vi "SSL Vision Log Player.vi"() -> ()   [LabVIEW 2017]
uses:
  SSL Referee Game Status.ctl
  GUI/IA Robot Line Display.ctl
  Intel/Functions Enum.ctl
  Filters/Estimadores.ctl
  Control/SSL Data Control.ctl
  Control/SSL UDP Address.ctl
  Control/File Player.ctl
  Intel/Command Enum.ctl
  Test/TestModule.ctl
  Util/Select None or Robot.ctl
  DrawTargets.ctl
  Select Personalitys.ctl
  Util/Select Auto None or Robot.ctl
  Intel/AI Parameters.ctl
  grSim/grSim RobotReplacement.ctl
  grSim/grSim_BallReplacement.ctl
  SSL/SSL Field State.ctl
  SSL Detection Frame.ctl
  SSL Detection Robot.ctl
  <vilib>/Analysis/Matrix/Datatypes/RealMatrix.ctl
  SSL Detection Ball.ctl
  <extravilib>/ChannelInstances/Lossy Stream-t'AI Input.ctl'/Read With Abort.vi
  <extravilib>/ChannelInstances/Lossy Stream-a[.](u8)/Read With Abort.vi
  <extravilib>/ChannelInstances/Lossy Stream-t'SSL Referee Game Status.ctl'/Write With Abort.vi
  <extravilib>/ChannelInstances/Lossy Stream-t'SSL Field State.ctl'/Write With Abort.vi
  <extravilib>/ChannelInstances/Lossy Stream-t'SSL Field State.ctl'/Read With Abort.vi
  <extravilib>/ChannelInstances/Lossy Stream-a[.](i32)/Write With Abort.vi
  <extravilib>/ChannelInstances/Lossy Stream-t'SSL Referee Game Status.ctl'/Read With Abort.vi
  <extravilib>/ChannelInstances/Lossy Stream-t'AI Input.ctl'/Write With Abort.vi
  <extravilib>/ChannelInstances/Lossy Stream-t'AI Input.ctl'/EndpointRead.vi
  <extravilib>/ChannelInstances/Lossy Stream-a[.](u8)/EndpointRead.vi
  <extravilib>/ChannelInstances/Lossy Stream-t'SSL Referee Game Status.ctl'/Endpoint.vi
  <extravilib>/ChannelInstances/Lossy Stream-t'SSL Field State.ctl'/Endpoint.vi
  <extravilib>/ChannelInstances/Lossy Stream-t'SSL Field State.ctl'/EndpointRead.vi
  <extravilib>/ChannelInstances/Lossy Stream-a[.](i32)/Endpoint.vi
  <extravilib>/ChannelInstances/Lossy Stream-t'SSL Referee Game Status.ctl'/EndpointRead.vi
  <extravilib>/ChannelInstances/Lossy Stream-t'AI Input.ctl'/Endpoint.vi
  <extravilib>/ChannelInstances/Lossy Stream-a[.](u8)/Instantiate.vi
  <extravilib>/ChannelInstances/Lossy Stream-a[.](u8)/)Channel.vi
  <resource>/ChannelSupport/_ChannelSupport/WaitIfNeeded.vi
  <extravilib>/ChannelInstances/Lossy Stream-t'AI Input.ctl'/Instantiate.vi
  <extravilib>/ChannelInstances/Lossy Stream-t'SSL Field State.ctl'/Instantiate.vi
  <extravilib>/ChannelInstances/Lossy Stream-t'AI Input.ctl'/)Channel.vi
  <extravilib>/ChannelInstances/Lossy Stream-t'SSL Field State.ctl'/)Channel.vi
  <extravilib>/ChannelInstances/Lossy Stream-a[.](i32)/Instantiate.vi
  Util/PreviousState.vi
  <extravilib>/ChannelInstances/Lossy Stream-t'SSL Referee Game Status.ctl'/Instantiate.vi
  <extravilib>/ChannelInstances/Lossy Stream-t'SSL Referee Game Status.ctl'/)Channel.vi
  <extravilib>/ChannelInstances/Lossy Stream-a[.](i32)/)Channel.vi
  <extravilib>/ChannelInstances/Lossy Stream-t'SSL Referee Game Status.ctl'.lvlib
  <extravilib>/ChannelInstances/Lossy Stream-t'AI Input.ctl'.lvlib
  <extravilib>/ChannelInstances/Lossy Stream-t'SSL Field State.ctl'.lvlib
  <extravilib>/ChannelInstances/Lossy Stream-a[.](u8).lvlib
  <vilib>/Analysis/Matrix/NI_Matrix.lvlib
  <extravilib>/ChannelInstances/Lossy Stream-a[.](i32).lvlib
panel:
  out "error IO":errorcluster
  out "Vector Flags":cluster{"id":dbl, "flag":bool}[](array[cluster])
  in  "grid y":dbl format="%#_13g"
  in  "grid x":dbl format="%#_13g"
  out "kick error":dbl
  in  "Pinned":T1={"Attc"="Auto", "Strk"="Auto", "Def"="Auto"}
  in  "Draw Targets?":T3={"Attacker"=TRUE, "Striker"=TRUE, "Goalie"=TRUE, "Defender"=TRUE, "kick"=TRUE, "Est Ball"=TRUE, "Est Robot"=FALSE}
  in  "SSL Data":T4={"Modo"=TRUE, "SSL UDP RX"={"Port:"=10020, "Server IP:"="224.5.23.2", "Local IP:"="", "RX"=TRUE}, "RefBox UDP RX"={"Port:"=10003, "Server IP:"="224.5.23.1", "Local IP:"="", "RX"=TRUE}, "Reprodução de Arquivo"={"file path (use dialog)"=path "E:/Media/2016-07-01_cmdragons_immortals.log", "size (in bytes)"=0, "offset (in bytes)"=0, "Slide"=0.0, "Play"=FALSE, "Time Stamp"=timestamp(0 s since 1904-01-01), "Playing"=FALSE}, "SSL UDP SOS RX "={"Port:"=10030, "Server IP:"="224.5.23.2", "Local IP:"="", "RX"=TRUE}} {"Reprodução de Arquivo"."Time Stamp" format="%<%.3X %x>T"; "Reprodução de Arquivo"."Slide" min=0 max=1 scale=0.0..1.0; "Reprodução de Arquivo"."offset (in bytes)" format="%.3p"; "Reprodução de Arquivo"."size (in bytes)" format="%.3p"}
  out "error out 5":errorcluster
  out "error out 3":errorcluster
  out "Pass":bool
  out "IA command":T7
  in  "ignora esquerda?":bool
  in  "ignora lado?":bool
  in  "atacando ao contrário?":bool
  in  "Defense stretch":i32=300
  in  "Defense radius":i32=460
  in  "Estimador":T8=enum."Kalman"
  out "Role Playing \nFPS":dbl
  out "Total Delay":dbl format="%#.5g"
  in  "Goalie":string(combo)="0"
  in  "Command":string(combo)="Auto"
  in  "Time":enum16{"Azul", "Amarelo"}(ring) caption="Enum"
  in  "Lado":enum16{"Esquerdo", "Direito"}(ring) caption="Enum"
  in  "Role Decisor":enum16{"Simple Role Decisor", "No Role Decisor"}(ring)
  out "bot velocity":dbl(graph)
  out "ball":dbl(graph)
  in  "test module":T9={"Goto"="None", "ZigZag 0"="None", "Kicker"="None", "Vel_kick"=100.0, "Kick"=FALSE, "Modo Teste?"=FALSE, "GoTo point"=[], "zigzag points"=[{"x"=666.0, "y"=0.0}, {"x"=-666.0, "y"=0.0}], "robot id vel"=5, "Dribble"=FALSE, "Gravando"=FALSE, "output xy"=0.0, "output angle"=0.0, "angle zigzag"=0.0}
  in  "Tab Control":enum32{"RX Info", "TX info", "AI Parameters"}(tab)
  out "GUI Robot Array":T11[](array[typedef])
  out "Game Status":T13={"Stage"="Normal First Half Pre", "Command"="Stop", "Time Left"=0.0, "Yellow Team"="", "Blue Team"="", "Yellow Score"=0, "Blue Score"=0, "Yellow Red Cards"=0, "Blue Red Cards"=0, "Yellow Yellow Cards"=0, "Blue Yellow Cards"=0, "Yellow Timeouts Left"=0, "Blue Timeouts Left"=0, "Yellow Timeout Remaining"=0.0, "Blue Timeout Remaining"=0.0, "Yellow Goalie Id"=0, "Blue Goalie Id"=0, "Time"=timestamp(2082758400 s since 1904-01-01)} {"Time" format="%<%.3X %x>T"; "Blue Timeout Remaining" format="%<%M:%S>t"; "Yellow Timeout Remaining" format="%<%M:%S>t"; "Time Left" format="%<%M:%S>t"}
  in  "Serial TX":bool
  in  "UDP TX":bool=TRUE
  in  "Address:":string="127.0.0.1"
  in  "Port:":u16=20011
  in  "Porta:":refnum<visa-resource-name>
  out "Comm FPS":dbl
  in  "replace active":bool
  in  "grSim replacement":cluster{"robots":T14[], "ball":T15}={"robots"=[{"x"=0.0, "y"=-450.0, "dir"=0.0, "yellowteam"=FALSE, "id"=0}, {"x"=0.0, "y"=-270.0, "dir"=0.0, "yellowteam"=FALSE, "id"=1}, {"x"=0.0, "y"=-90.0, "dir"=0.0, "yellowteam"=FALSE, "id"=2}, {"x"=0.0, "y"=90.0, "dir"=0.0, "yellowteam"=FALSE, "id"=3}, {"x"=0.0, "y"=270.0, "dir"=0.0, "yellowteam"=FALSE, "id"=4}, {"x"=0.0, "y"=450.0, "dir"=0.0, "yellowteam"=FALSE, "id"=5}], "ball"={"x"=0.0, "y"=0.0, "vx"=0.0, "vy"=0.0}}
  in  "AI Parameters":T16={"GotoKick"={"Dist do cone a frente"=0.0, "attacker farback"=1000.0, "Perto"=300.0, "min dist to kick"=120.0, "kick eps"=0.1, "Time to transition"=0.3}, "Attacker"={"CC chute"=0.55, "CC passe"=0.4, "Kick Force"=100.0, "D ball-robot Kick"=250.0, "D ball-robot Pass"=350.0}, "Defender"={"D max"=1700.0, "Vel p/ robô av"=3.0, "Kick Force"=100.0, "D atk-def"=400.0, "D farback"=300.0}, "Timeout"={"Field/v in x"=6.0, "Dist Robots"=300, "Dist up in y"=300}, "Pose Striker"={"dist"=650.0, "Numeric"=-4.0, "dist 2"=650.0}, "Dist Stop"=300.0, "Distance when ball out"=200, "D central gap "=125.0, "T pass"=5.0, "Force ++"=100.0, "range kick"=50.0, "Chute alto"=TRUE, "Marcador novo"=TRUE} {"D central gap" format="%#_13g"; "Dist Stop" format="%#_13g"; "Pose Striker"."Numeric" format="%#_13g"; "Defender"."Kick Force" format="%#_13g"; "Defender"."Vel p/ robô av" format="%#_13g"; "Attacker"."D ball-robot Kick" format="%#_13g"; "Attacker"."Kick Force" format="%#_13g"; "Attacker"."CC passe" format="%#_13g"; "Attacker"."CC chute" format="%#_13g"; "GotoKick"."min dist to kick" format="%#_13g"; "GotoKick"."Perto" format="%#_13g"; "GotoKick"."attacker farback" format="%#_13g"; "GotoKick"."Dist do cone a frente" format="%#_13g"}
  in  "Dist posse":dbl=220.0
  in  "Tol ang posse":dbl=0.3
  in  "Dist Toque":dbl=130.0
  in  "Qtd Min p/ Stk":dbl=2.0
  # "UDP"
  # "LOG"
  # "Score"
  # "Red Cards"
  # "Yellow Cards"
  # "Timeouts Left"
  # "Timeout Remaining"
  # "Goalie ID"
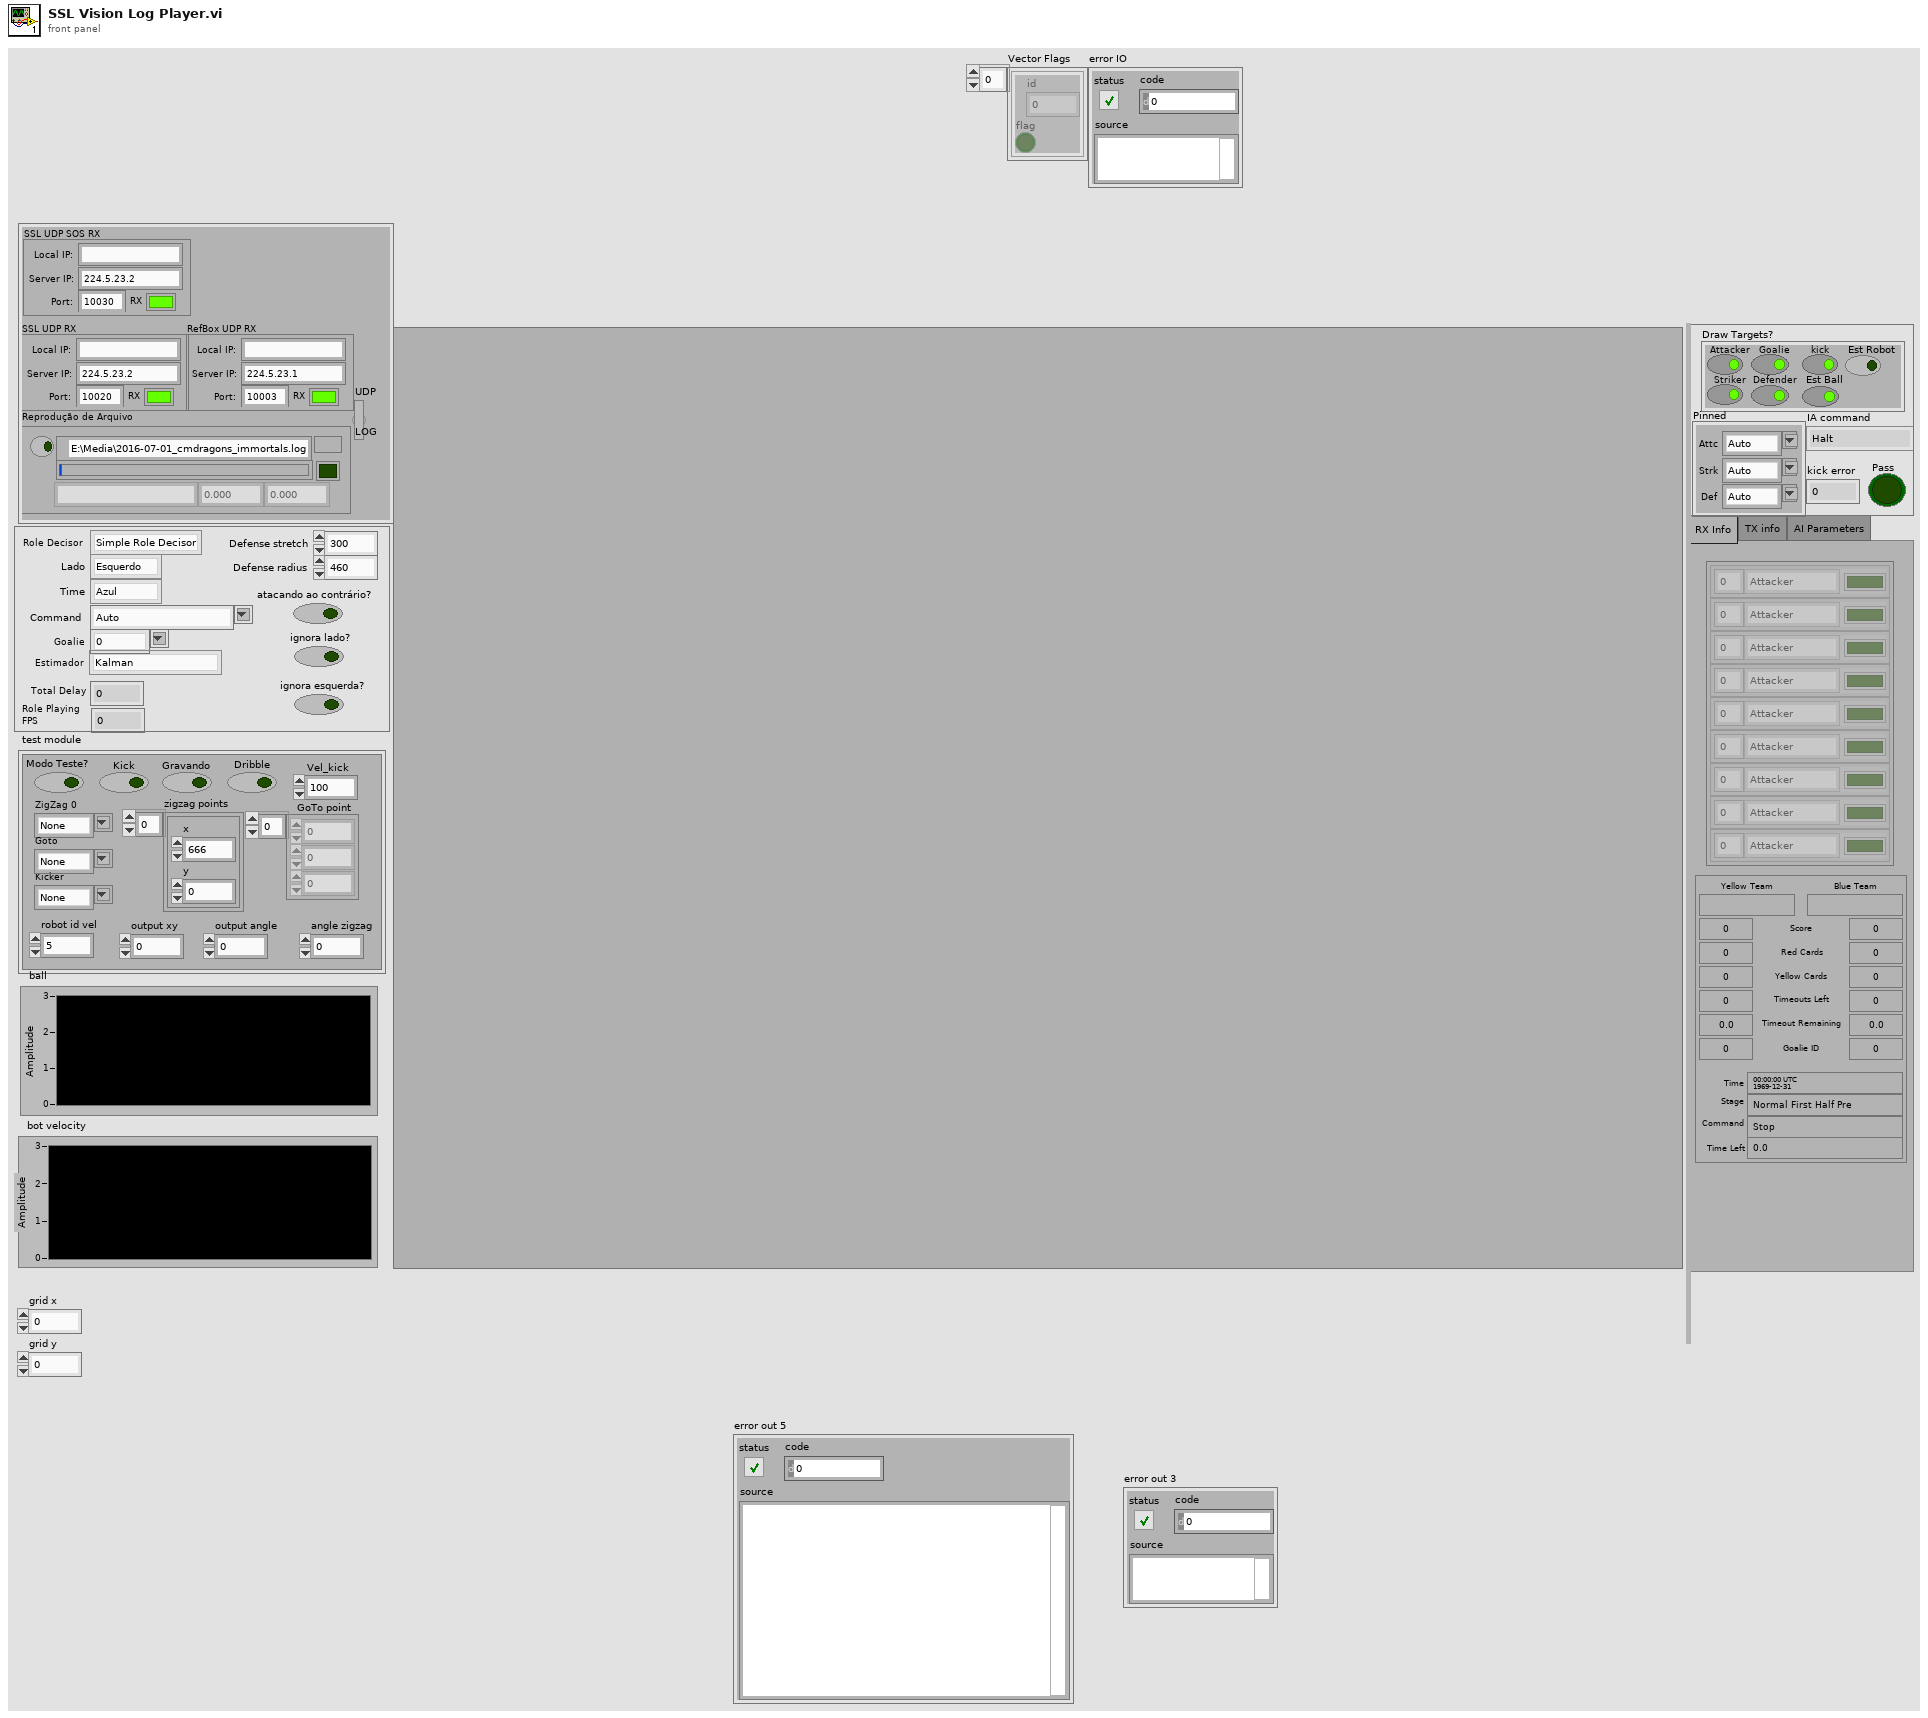
[diagram p1: front panel]
types:
  T1 = typedef "Select Personalitys.ctl" = cluster{"Attc":T2, "Strk":T2, "Def":T2}
  T2 = typedef "Select Auto None or Robot.ctl" = string
  T3 = typedef "DrawTargets.ctl" = cluster{"Attacker":bool, "Striker":bool, "Goalie":bool, "Defender":bool, "kick":bool, "Est Ball":bool, "Est Robot":bool}
  T4 = typedef "SSL Data Control.ctl" = cluster{"Modo":bool, "SSL UDP RX":T5, "RefBox UDP RX":T5, "Reprodução de Arquivo":T6, "SSL UDP SOS RX ":T5}
  T5 = typedef "SSL UDP Address.ctl" = cluster{"Port:":u16, "Server IP:":string, "Local IP:":string, "RX":bool}
  T6 = typedef "File Player.ctl" = cluster{"file path (use dialog)":path, "size (in bytes)":i64, "offset (in bytes)":i64, "Slide":sgl, "Play":bool, "Time Stamp":timestamp, "Playing":bool}
  T7 = typedef "Command Enum.ctl" = enum16{"Halt", "Stop", "Force Start", "PKA Normal Start", "Prepare Kickoff Ally", "PKE Normal Start", "Prepare Kickoff Enemy", "Prepare Penalty Ally", "PPA Normal Start", "Prepare Penalty Enemy", "PPE Normal Start", "Direct Free Enemy", "Direct Free Ally", "Indirect Free Enemy", "Indirect Free Ally", "Timeout Enemy", "Timeout Ally", "Goal Enemy", "Goal Ally", "Ball Placement Enemy", "Ball Placement Ally", "Normal Half Time", "Extra Time Break", "Extra Half Time", "None", "Post Game"}
  T8 = typedef "Estimadores.ctl" = enum16{"Nenhum", "Simples", "Kalman"}
  T9 = typedef "TestModule.ctl" = cluster{"Goto":T10, "ZigZag 0":T10, "Kicker":T10, "Vel_kick":dbl, "Kick":bool, "Modo Teste?":bool, "GoTo point":dbl[], "zigzag points":cluster{"x":dbl, "y":dbl}[], "robot id vel":u32, "Dribble":bool, "Gravando":bool, "output xy":dbl, "output angle":dbl, "angle zigzag":dbl}
  T10 = typedef "Select None or Robot.ctl" = string
  T11 = typedef "IA Robot Line Display.ctl" = cluster{"ID":dbl, "function":T12, "dribble":bool}
  T12 = typedef "Functions Enum.ctl" = enum16{"Attacker", "Goalie", "Defender", "Striker", "Goto 0", "Dummy", "Kicker", "ZigZag"}
  T13 = typedef "SSL Referee Game Status.ctl" = cluster{"Stage":string, "Command":string, "Time Left":dbl, "Yellow Team":string, "Blue Team":string, "Yellow Score":u32, "Blue Score":u32, "Yellow Red Cards":u32, "Blue Red Cards":u32, "Yellow Yellow Cards":u32, "Blue Yellow Cards":u32, "Yellow Timeouts Left":u32, "Blue Timeouts Left":u32, "Yellow Timeout Remaining":dbl, "Blue Timeout Remaining":dbl, "Yellow Goalie Id":u32, "Blue Goalie Id":u32, "Time":timestamp}
  T14 = typedef "grSim RobotReplacement.ctl" = cluster{"x":dbl, "y":dbl, "dir":dbl, "yellowteam":bool, "id":u32}
  T15 = typedef "grSim_BallReplacement.ctl" = cluster{"x":dbl, "y":dbl, "vx":dbl, "vy":dbl}
  T16 = typedef "AI Parameters.ctl" = cluster{"GotoKick":cluster{"Dist do cone a frente":dbl, "attacker farback":dbl, "Perto":dbl, "min dist to kick":dbl, "kick eps":dbl, "Time to transition":dbl}, "Attacker":cluster{"CC chute":dbl, "CC passe":dbl, "Kick Force":dbl, "D ball-robot Kick":dbl, "D ball-robot Pass":dbl}, "Defender":cluster{"D max":dbl, "Vel p/ robô av":dbl, "Kick Force":dbl, "D atk-def":dbl, "D farback":dbl}, "Timeout":cluster{"Field/v in x":dbl, "Dist Robots":u32, "Dist up in y":u32}, "Pose Striker":cluster{"dist":dbl, "Numeric":dbl, "dist 2":dbl}, "Dist Stop":dbl, "Distance when ball out":i32, "D central gap ":dbl, "T pass":dbl, "Force ++":dbl, "range kick":dbl, "Chute alto":bool, "Marcador novo":bool}
  T17 = typedef "Lossy Stream-a[.](u8).lvlib/)Channel.ctl" = refnum<queue>
  T18 = typedef "SSL Field State.ctl" = cluster{"Detection Frame Out":T19, "Field Size Out":cluster{"line_width":u32, "field_length":u32, "field_width":u32, "boundary_width":u32, "referee_width":u32, "goal_width":u32, "goal_depth":u32, "goal_wall_width":u32, "center_circle_radius":u32, "defense_radius":u32, "defense_stretch":u32, "free_kick_from_defense_dist":u32, "penalty_spot_from_field_line_dist":u32, "penalty_line_from_spot_dist":u32}, "Received Time Stamp":timestamp}
  T19 = typedef "SSL Detection Frame.ctl" = cluster{"frame_number":u32, "t_capture":dbl, "t_sent":dbl, "camera_id":u32, "robots_yellow":T20[], "robots_blue":T20[], "balls":T22[], "Valid":bool, "Time Stamp":timestamp}
  T20 = typedef "SSL Detection Robot.ctl" = cluster{"x":sgl, "robot_id":u32, "confidence":sgl, "y":sgl, "orientation":sgl, "pixel_x":sgl, "pixel_y":sgl, "height":sgl, "Valid":bool, "Time Stamp":timestamp, "x_k|k":T21, "Pk|k":T21, "Previous Time Stamp":timestamp, "R":T21}
  T21 = typedef "NI_Matrix.lvlib/RealMatrix.ctl" = dbl[][]
  T22 = typedef "SSL Detection Ball.ctl" = cluster{"x":sgl, "area":u32, "confidence":sgl, "y":sgl, "z":sgl, "pixel_x":sgl, "pixel_y":sgl, "Valid":bool, "Time Stamp":timestamp, "x_k|k":T21, "Pk|k":T21, "Id":u32, "Previous Time Stamp":timestamp, "R":T21}
  T23 = cluster{"line_width":u32, "field_length":u32, "field_width":u32, "boundary_width":u32, "referee_width":u32, "goal_width":u32, "goal_depth":u32, "goal_wall_width":u32, "center_circle_radius":u32, "defense_radius":u32, "defense_stretch":u32, "free_kick_from_defense_dist":u32, "penalty_spot_from_field_line_dist":u32, "penalty_line_from_spot_dist":u32}
  T24 = typedef "Lossy Stream-t'SSL Field State.ctl'.lvlib/)Channel.ctl" = refnum<queue>
  T25 = typedef "SSL Referee.ctl" = cluster{"packet_\ntimestamp":u64, "stage":u64, "stage_time_left":i32, "command ":u64, "command_\ncounter ":u32, "command_\ntimestamp":u64, "yellow team info":T26, "blue team info":T26, "Point":cluster{"x":sgl, "y":sgl}}
  T26 = typedef "SSL Referee Team Info.ctl" = cluster{"name":string, "score":u32, "red_cards":u32, "yellow_cards_time":u32[], "yellow_cards":u32, "timeout":u32, "timeout_times":u32, "goalie":u32}
  T27 = typedef "Lossy Stream-t'SSL Referee Game Status.ctl'.lvlib/)Channel.ctl" = refnum<queue>
  T28 = typedef "AI Input.ctl" = cluster{"our_robots":T29[], "enemy_robots":T29[], "balls":T31[], "geometry":T32, "IA Judge":T33, "Received Timestamp":timestamp, "Events":T34}
  T29 = typedef "AI Robot.ctl" = cluster{"id":u32, "function":T12, "x":dbl, "y":dbl, "orientation":dbl, "v_tangent":dbl, "v_normal":dbl, "v_ang":dbl, "kick_x":dbl, "kick_z":dbl, "dribble":bool, "Timestamp":timestamp, "dest_x":dbl, "dest_y":dbl, "dest_orientation":dbl, "estimatives":cluster{"est_v_tangent":dbl, "est_v_normal":dbl, "est_vx":dbl, "est_vy":dbl, "Pos Robot Est":dbl[]}, "dest_x_kick":dbl, "dest_y_kick":dbl, "Gap Coord":dbl[], "States":T30}
  T30 = typedef "AttackerStates.ctl" = enum16{"Pass", "GoToTangent", "BallGetting", "GoToKick", ""}
  T31 = typedef "AI Ball.ctl" = cluster{"x":dbl, "y":dbl, "timestamp":timestamp, "Vel_x":dbl, "Vel_y":dbl, "Pos Bola Est":dbl[]}
  T32 = typedef "Field Size.ctl" = cluster{"line_width":u32, "field_length":u32, "field_width":u32, "boundary_width":u32, "referee_width":u32, "goal_width":u32, "goal_depth":u32, "goal_wall_width":u32, "center_circle_radius":u32, "defense_radius":u32, "defense_stretch":u32, "free_kick_from_defense_dist":u32, "penalty_spot_from_field_line_dist":u32, "penalty_line_from_spot_dist":u32}
  T33 = typedef "AI Judge.ctl" = cluster{"stage":string, "command":string, "our_goalie_id":dbl, "enemy_goalie_id":dbl, "command enum":T7, "Time":enum16{"Azul", "Amarelo"}}
  T34 = typedef "Events.ctl" = cluster{"Touch":bool, "Ball out":bool, "id touch":dbl, "Ball out of \nVision":bool, "Ball inside \nGoalie area":bool, "Robot not responding":bool, "Robots responding status":dbl[], "Enemy Ball \nPossession":bool, "Pass State":bool, "id end of pass":dbl, "Kick":bool, "Id ini Possession":dbl, "Ball Possesion":bool, "Id Possesion":dbl}
  T35 = typedef "Lossy Stream-a[.](i32).lvlib/)Channel.ctl" = refnum<queue>
  T36 = typedef "Lossy Stream-t'AI Input.ctl'.lvlib/)Channel.ctl" = refnum<queue>
  T37 = typedef "grSim Robot Command.ctl" = cluster{"id":u32, "kickspeedx":sgl, "kickspeedz":sgl, "veltangent":sgl, "velnormal":sgl, "velangular":sgl, "spinner":bool, "wheelspeed":bool, "wheel1":sgl, "wheel2":sgl, "wheel3":sgl, "wheel4":sgl}
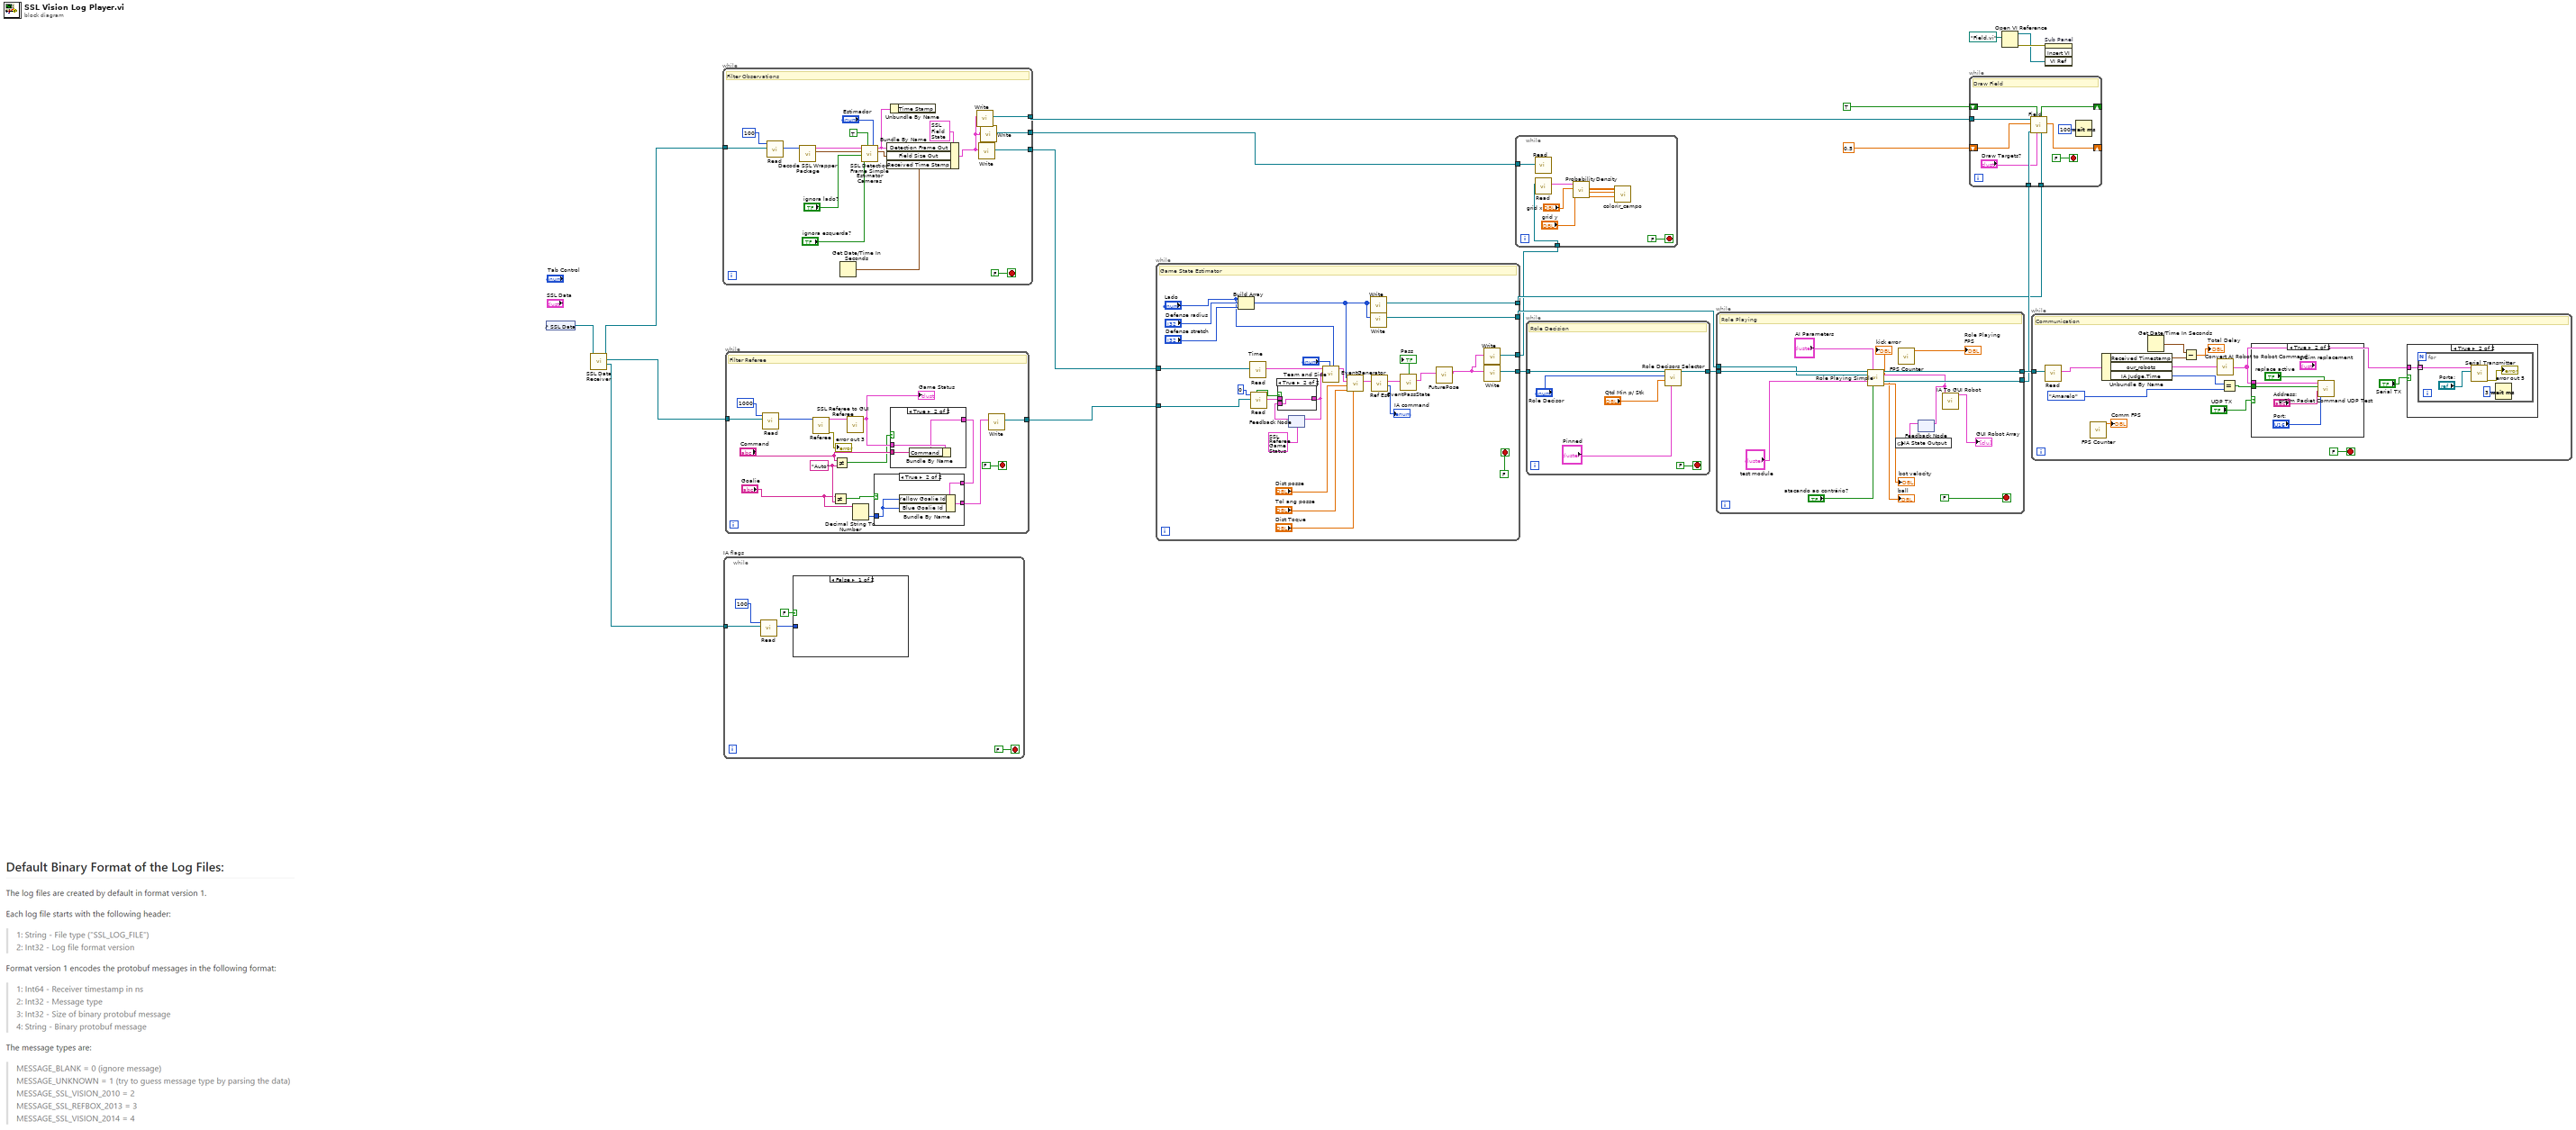
[diagram p0: block diagram]
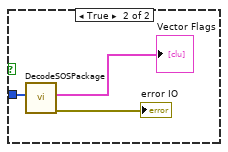
[diagram p2: hidden frame]
diagram:
  n1 = control-ref of="SSL Data"() -> (w2:refnum<vi>)
  n2 = call "SSL Data Receiver.vi"("SSL Data 2"=w2) -> ("IA flags"=w1:T17, "SSL RefBox"=w11:T17, "SSL Vision"=w12:T17)  [unwired: 8 in]
  n3 = while {
    tunnel: [w23] -> w9
    tunnel: [w31] -> w15
    tunnel: w12 -> [w28]
    tunnel: [w21] -> w4
    stop <- FALSE stop-if-true
    # "Filter Observations"
    n4 = call <extravilib>:"Read.vi"("channel"=w28, "timeout in ms (-1)"=100) -> ("element"=w27:u8[])  [unwired: 4 in, 5 out]
    n5 = call "Decode SSL Wrapper Package.vi"("unsigned byte array"=w27) -> ("Field Size"=w36:T23, "Detection Frame"=w37:T19)  [unwired: 7 in, 2 out]
    n6 = Get Date/Time In Seconds() -> (seconds since 1Jan1904=w33:timestamp)
    n7 = call "SSL Detection Frame Simple Estimator Cameras.vi"("Estimador"="Estimador", "Enable"=TRUE, "ignora esquerda?"="ignora esquerda?", "ignora lado?"="ignora lado?", "Field Size"=w36, "Detection Frame In"=w37) -> ("Field Size Out"=w32:T23, "Detection Frame Out"=w30:T19)  [unwired: 4 in]
    n8 = Bundle By Name(cluster=T18 {"Detection Frame Out"={"frame_number"=0, "t_capture"=0.0, "t_sent"=0.0, "camera_id"=0, "robots_yellow"=[], "robots_blue"=[], "balls"=[], "Valid"=FALSE, "Time Stamp"=timestamp(0 s since 1904-01-01)}, "Field Size Out"={"line_width"=0, "field_length"=0, "field_width"=0, "boundary_width"=0, "referee_width"=0, "goal_width"=0, "goal_depth"=0, "goal_wall_width"=0, "center_circle_radius"=0, "defense_radius"=0, "defense_stretch"=0, "free_kick_from_defense_dist"=0, "penalty_spot_from_field_line_dist"=0, "penalty_line_from_spot_dist"=0}, "Received Time Stamp"=timestamp(0 s since 1904-01-01)}, "Detection Frame Out"=w30, "Field Size Out"=w32, "Received Time Stamp"=w33) -> (w22:T18)
    n9 = Unbundle By Name(w30) -> ()  [unwired: 1 out]
    n10 = call <extravilib>:"Write.vi"("element"=w22) -> ("channel"=w23:T24)  [unwired: 8 in, 2 out]
    n11 = call <extravilib>:"Write.vi"("element"=w22) -> ("channel"=w31:T24)  [unwired: 8 in, 2 out]
    n12 = call <extravilib>:"Write.vi"("element"=w22) -> ("channel"=w21:T24)  [unwired: 8 in, 2 out]
  }
  n13 = while "IA flags" {
    tunnel: w1 -> [w42]
    stop <- FALSE stop-if-true
    n14 = call <extravilib>:"Read.vi"("channel"=w42, "timeout in ms (-1)"=100) -> ("element"=w41:u8[])  [unwired: 4 in, 5 out]
    n15 = case shown="False" FALSE {
      tunnel: w41 -> [_ w46]
      frame False {
      }
      frame True {
        n16 = call "DecodeSOSPackage.vi"("Array"=w46) -> ("error IO"=→"error IO":errorcluster, "Vector Flags"=→"Vector Flags":cluster{"id":dbl, "flag":bool}[])  [unwired: 9 in]
      }
    }
  }
  n17 = while {
    tunnel: w11 -> [w49]
    tunnel: [w59] -> w14
    stop <- FALSE stop-if-true
    w55 = "Auto" ("y")
    # "Filter Referee"
    n18 = call <extravilib>:"Read.vi"("channel"=w49, "timeout in ms (-1)"=1000) -> ("element"=w48:u8[])  [unwired: 4 in, 5 out]
    n19 = call "Referee.vi"("element"=w48) -> ("output cluster"=w60:T25, "error out"=→"error out 3":errorcluster)  [unwired: 13 in]
    n20 = Not Equal?(x="Goalie", y=w55) -> (x != y?=w54:bool)
    n21 = Not Equal?(x="Command", y=w55) -> (x != y?=w56:bool)
    n22 = call "SSL Referee to GUI Referee.vi"("SSL Game Status"=w60) -> ("GUI Game Status"=w58:T13)  [unwired: 10 in]
    "Game Status" <- w58
    n23 = Decimal String To Number(string="Goalie") -> (number=w50:i32)  [unwired: 2 in, 1 out]
    n24 = case shown="True" w56 {
      tunnel: w58 -> [w67 w70]
      tunnel: [w67 w69] -> w53
      tunnel: "Command" -> [_ w68]
      frame False {
      }
      frame True {
        n25 = Bundle By Name(cluster=w70, "Command"=w68) -> (w69:T13)
      }
    }
    n26 = case shown="True" w54 {
      tunnel: w53 -> [w63 w66]
      tunnel: [w63 w65] -> w52
      tunnel: w50 -> [_ w64]
      frame False {
      }
      frame True {
        n27 = Bundle By Name(cluster=w66, "Yellow Goalie Id"=w64, "Blue Goalie Id"=w64) -> (w65:T13)
      }
    }
    n28 = call <extravilib>:"Write.vi"("element"=w52) -> ("channel"=w59:T27)  [unwired: 8 in, 2 out]
  }
  n29 = while {
    tunnel: w15 -> [w89]
    tunnel: w14 -> [w98]
    tunnel: [w92] -> w10
    tunnel: [w82] -> w5
    tunnel: [w80] -> w6
    tunnel: [w71] -> w3
    stop <- FALSE stop-if-true
    # "Game State Estimator"
    n30 = Build Array("Lado", "Defense radius", "Defense stretch") -> (w81:i32[])
    n31 = call <extravilib>:"Read.vi"("channel"=w89) -> ("element"=w88:T18)  [unwired: 5 in, 5 out]
    n32 = call <extravilib>:"Read.vi"("channel"=w98, "timeout in ms (-1)"=0) -> ("element"=w95:T13, "timed out?"=w96:bool)  [unwired: 4 in, 4 out]
    n33 = feedback #1(T13 {"Stage"="First Half", "Command"="Stop", "Time Left"=0.0, "Yellow Team"="", "Blue Team"="", "Yellow Score"=0, "Blue Score"=0, "Yellow Red Cards"=0, "Blue Red Cards"=0, "Yellow Yellow Cards"=0, "Blue Yellow Cards"=0, "Yellow Timeouts Left"=0, "Blue Timeouts Left"=0, "Yellow Timeout Remaining"=0.0, "Blue Timeout Remaining"=0.0, "Yellow Goalie Id"=0, "Blue Goalie Id"=0, "Time"=timestamp(0 s since 1904-01-01)} ("element")) -> (w94:T13)
    n34 = case shown="True" w96 {
      tunnel: w95 -> [w100 _]
      tunnel: [w100 w101] -> w93
      tunnel: w94 -> [_ w101]
      frame False {
      }
      frame True {
      }
    }
    n35 = feedback-in #1(w93) -> ()
    n36 = call "Team and Side.vi"("Lado"="Lado", "Time"="Time", "Game Status"=w93, "Field State Input"=w88) -> ("IA State"=w87:T28)  [unwired: 7 in]
    n37 = call "EventGenerator.vi"("Dist Para Toque"="Dist Toque", "Tol para ang posse"="Tol ang posse", "Dist Para posse"="Dist posse", "IA State Input"=w87, "lado, readius, stretch"=w81) -> ("IA State Output"=w86:T28)  [unwired: 6 in]
    n38 = call <extravilib>:"Write.vi"("element"=w81) -> ("channel"=w80:T35)  [unwired: 8 in, 2 out]
    n39 = call <extravilib>:"Write.vi"("element"=w81) -> ("channel"=w82:T35)  [unwired: 8 in, 2 out]
    n40 = call "Ref Est.vi"("IA State Input"=w86) -> ("IA command"=→"IA command":T7, "IA State Output"=w78:T28)  [unwired: 9 in]
    n41 = call "EventPassState.vi"("IA State Input"=w78) -> ("IA State Output"=w76:T28, "Pass State"=→"Pass":bool)  [unwired: 8 in, 1 out]
    n42 = call "FuturePose.vi"("IA State Input"=w76) -> ("output cluster"=w72:T28)  [unwired: 10 in]
    n43 = call <extravilib>:"Write.vi"("element"=w72) -> ("channel"=w71:T36)  [unwired: 8 in, 2 out]
    n44 = call <extravilib>:"Write.vi"("element"=w72) -> ("channel"=w92:T36)  [unwired: 8 in, 2 out]
  }
  n45 = while {
    tunnel: w4 -> [w109]
    tunnel: w3 -> [w108]
    stop <- FALSE stop-if-true
    n46 = call <extravilib>:"Read.vi"("channel"=w109) -> ()  [unwired: 5 in, 6 out]
    n47 = call <extravilib>:"Read.vi"("channel"=w108) -> ("element"=w107:T28)  [unwired: 5 in, 5 out]
    n48 = call "ProbabilityDensity.vi"("grid y"="grid y", "grid x"="grid x", "IA state"=w107) -> ("grid y out"=w102:dbl, "grid x out"=w103:dbl, "3D Probability Matrix"=w104:dbl[][][])  [unwired: 6 in]
    n49 = call "colorir_campo.vi"("grid y"=w102, "grid x"=w103, "3D Probability Matrix"=w104) -> ()  [unwired: 9 in]
  }
  n50 = while {
    tunnel: w10 -> [w114]
    tunnel: [w113] -> w8
    stop <- FALSE stop-if-true
    # "Role Decision"
    n51 = call "Role Decisors Selector.vi"("Pinned"="Pinned", "Qtd Min p/ Stk"="Qtd Min p/ Stk", "Role Decisor"="Role Decisor", "channel"=w114) -> ("channel"=w113:T36)  [unwired: 6 in, 1 out]
  }
  n52 = while {
    tunnel: w8 -> [w130]
    tunnel: [w129] -> w13
    tunnel: [w125] -> w7
    tunnel: w6 -> [w124]
    stop <- FALSE stop-if-true
    # "Role Playing"
    n53 = call "Role Playing Simple.vi"(0:"channel"=w130, "AI Parameters"="AI Parameters", 5:"channel"=w124, "test module"="test module", "atacando ao contrário?"="atacando ao contrário?") -> ("kick \nerror"=→"kick error":dbl, "channel"=w129:T36, "IA State Output"=w119:T28, "channel to field"=w125:T36, "ball"=→"ball":dbl, "Robot"=→"bot velocity":dbl)  [unwired: 5 in]
    n54 = call "FPS Counter.vi"() -> ("Numeric"=→"Role Playing \nFPS":dbl)  [unwired: 11 in]
    n55 = feedback #2() -> (w120:T28)  [unwired: 1 in]
    n56 = global write "PreviousState.vi" "IA State Output"(w120) -> ()
    n57 = feedback-in #2(w119) -> ()
    n58 = call "IA To GUI Robot.vi"("Output IA"=w119) -> ("GUI Robot Array"=→"GUI Robot Array":T11[])  [unwired: 10 in]
  }
  n59 = while {
    shift-right: [w140] -> _
    shift-left: 0.5 ("New Scale") -> [w134]
    shift-right: [w139] -> _
    shift-left: TRUE ("AutoScale Out") -> [w138]
    tunnel: w7 -> [w136]
    tunnel: w9 -> [w135]
    tunnel: w5 -> [w133]
    stop <- FALSE stop-if-true
    # "Draw Field"
    n60 = call "Field.vi"("channel 2"=w133, "Draw Targets?"="Draw Targets?", "AutoScale"=w138, "channel for IA State"=w136, "Scale mm/pixel"=w134, "channel"=w135) -> ("Scale Out"=w140:dbl, "AutoScale Out"=w139:bool)  [unwired: 3 in, 1 out]
    n61 = Wait (ms)(milliseconds to wait=u32 100) -> ()  [unwired: 1 out]
  }
  n62 = Open VI Reference(vi path=path "Field.vi") -> (vi reference=w18:refnum<vi>, error out=w19:errorcluster)  [unwired: 5 in]
  n63 = while {
    tunnel: w13 -> [w154]
    stop <- FALSE stop-if-true
    # "Communication"
    n64 = call <extravilib>:"Read.vi"("channel"=w154) -> ("element"=w153:T28)  [unwired: 5 in, 5 out]
    n65 = call "FPS Counter.vi"() -> ("Numeric"=→"Comm FPS":dbl)  [unwired: 11 in]
    n66 = Unbundle By Name(w153) -> ("Received Timestamp"=w148:timestamp, "our_robots"=w152:T29[], "IA Judge.Time"=w151:enum16{"Azul", "Amarelo"})
    n67 = Get Date/Time In Seconds() -> (seconds since 1Jan1904=w147:timestamp)
    n68 = Subtract(x=w147, y=w148) -> (x-y=→"Total Delay":dbl)
    n69 = call "Convert AI Robot to Robot Command.vi"("Input Array"=w152) -> ("Output Array"=w145:T37[])
    n70 = Equal?(x=w151, y=enum16{"Azul", "Amarelo"}."Amarelo") -> (x = y?=w149:bool)
    n71 = case shown="True" "UDP TX" {
      tunnel: w149 -> [_ w165]
      tunnel: w145 -> [_ w163]
      frame False {
      }
      frame True {
        n72 = call "grSim Packet Command UDP Test.vi"("replace ball"="replace active", "Port:"="Port:", "SSL Vision Address:"="Address:", "isteamyellow"=w165, "Robots"=w163) -> ()  [unwired: 7 in]
      }
    }
    n73 = case shown="True" "Serial TX" {
      tunnel: w145 -> [_ w156]
      frame False {
      }
      frame True {
        n74 = for {
          tunnel: w156 -> [w160] mode=indexing
          n75 = call "Serial Transmitter.vi"("Porta:"="Porta:", "Robots"=w160) -> ("error out"=→"error out 5":errorcluster)  [unwired: 9 in]
          n76 = Wait (ms)(milliseconds to wait=u32 3) -> ()  [unwired: 1 out]
        }
      }
    }
  }
  n77 = invoke on="Sub Panel" class="SubPnl" method="Insert VI"(error in=w19, "VI Ref"=w18) -> ()  [unwired: 2 in, 4 out]
